vi "AI IRQ Config Pane.vi"(6 "_SubPanelMessages":refnum<notifier>, 9 "_myEmbeddedToFrameEvent":T7, 10 "_myEmbedded.Exit":refnum<user-event>, 11 "_Property Bundle":cluster{"Name":string, "Value":variant}[](array[cluster])) -> (1 "_Connection Informations":T2, 2 "_Scripter Input":T4)   [LabVIEW 2021]
doc: "Registers analog and digital input interrupts and creates timer interrupts."
uses:
  <vilib>/myRIO/Common/Express VI Framework/xctls/myRIO Channel Name/myRIO Channel Name.xctl
  <vilib>/myRIO/Common/Instrument Driver Framework/myRIO v1.0/IRQ/typedefs/AI IRQ Type.ctl
  <vilib>/myRIO/Common/Express VI Framework/typedefs/Config Pane to Framework Ref.ctl
  <vilib>/myRIO/Common/Express VI Framework/typedefs/Data Validate Ref.ctl
  <vilib>/myRIO/Common/Express VI Framework/typedefs/Sub Panel Messages.ctl
  <vilib>/myRIO/Common/Express VI Framework/typedefs/Instrument Driver Method Descriptor Array.ctl
  <vilib>/myRIO/Common/Express VI Framework/typedefs/Instrument Driver Method Descriptor.ctl
  <vilib>/myRIO/Common/Express VI Framework/typedefs/Scripter Input.ctl
  <vilib>/myRIO/Common/Express VI Framework/typedefs/WireThrough Terminal Names.ctl
  <vilib>/myRIO/Common/Express VI Framework/typedefs/Connection Informations.ctl
  <vilib>/myRIO/Common/Instrument Driver Framework/Utilities/typedefs/Channel Types.ctl
  <vilib>/myRIO/Common/Express VI Framework/vis/Express VI Framework Strings Global.vi
  <vilib>/myRIO/Express VI/IRQ/Message Globals.vi
panel:
  out "_create Callback?":bool
  in  "_Create Button":bool
  in  "Callback VI Path:":path
  out "_Warning Icon":picture
  out "_Error Message":string
  out "_Callback VI Path":string caption="Callback VI:"
  in  "_Open Button":bool
  out "_Hysteresis":string
  out "_Threhold":string
  out "_Analog Preview":T1(graph) caption="Preview:"
  in  "_callback":refnum<vi>
  in  "_VI Default Name (Edit and make value default)":string="Analog input interrupt"
  in  "_WireThrough Info (Edit and make value default)":T3={"WireThrough Top In"="Ref In", "WireThrough Bottom In"="error in (no error)", "WireThrough Top Out"="Ref Out", "WireThrough Bottom Out"="error out"}
  in  "_Template Array (Edit and make value default)":T5=[{"Function Name"="Register AI IRQ", "VI Path"=path "<vilib>/myRIO/Instrument Drivers/IRQ/IO IRQ/vis", "Script"=TRUE, "Inputs"=[{"name"="IRQ Number", "value"=variant, "Config Pane Only"=TRUE, "Build Array"=FALSE, "Bundle Cluster"=FALSE, "Show Term"=FALSE, "alias"=[], "Required Input"=FALSE}, {"name"="Analog Interrupt Type", "value"=variant, "Config Pane Only"=TRUE, "Build Array"=FALSE, "Bundle Cluster"=FALSE, "Show Term"=FALSE, "alias"=[], "Required Input"=FALSE}, {"name"="Channel Name", "value"=variant, "Config Pane Only"=TRUE, "Build Array"=FALSE, "Bundle Cluster"=FALSE, "Show Term"=FALSE, "alias"=[], "Required Input"=FALSE}, {"name"="Threshold", "value"=variant, "Config Pane Only"=TRUE, "Build Array"=FALSE, "Bundle Cluster"=FALSE, "Show Term"=FALSE, "alias"=[], "Required Input"=FALSE}, {"name"="Callback VI Reference", "value"=variant, "Config Pane Only"=FALSE, "Build Array"=FALSE, "Bundle Cluster"=FALSE, "Show Term"=TRUE, "alias"=[], "Required Input"=FALSE}], "Outputs"=[], "VI Class"=enum."Open", "Controls Refs[]"=[], "Inline"=FALSE}]
  in  "_Default Alias String":string
  in  "Type:":T9
  in  "Channel:":u16(xcontrol)
  in  "IRQ number:":u8 max=7
  in  "Threshold:":dbl=2.5 min=0.0 max=5.0
  in  "Name:":string="Analog input interrupt" caption="Node name:"
  out "_IRQ Learn More":string="The 0.02 hysteresis helps prevent multiple triggers due to noise."
  # "NOTE: Tab Order has been set\nfor this Front Panel.\n\nSee Edit>>Set Tabbing Order...\n\nAll controls that are not visible at \nruntime are excluded from Tabbing order\n\nTo exlude a control from context\nhelp prefix its label text with a '-'"
  # "Trigger point"
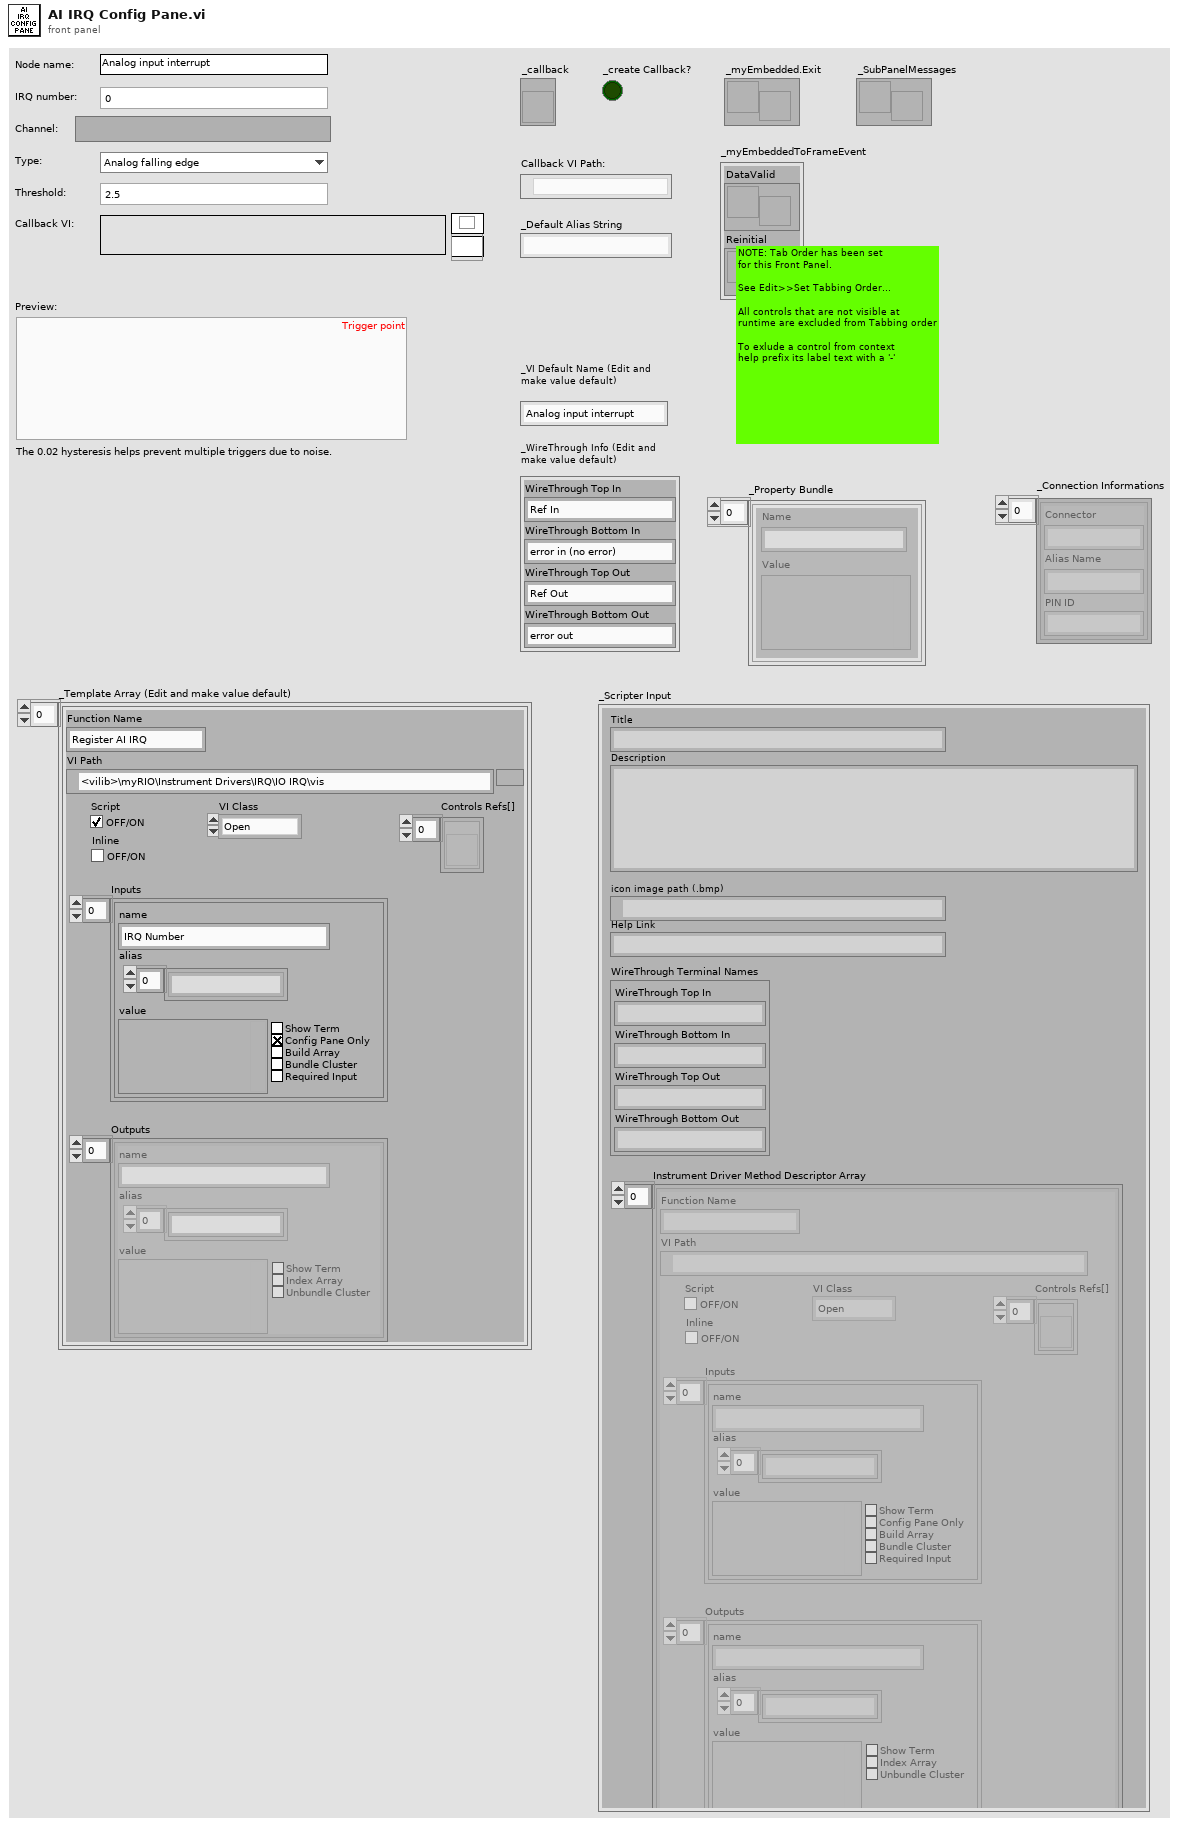
[diagram p1: front panel]
types:
  T1 = cluster{"Analog Preview 3":cluster{"X":dbl, "Y":dbl}[]}[]
  T2 = typedef "Connection Informations.ctl" = cluster{"Connector":string, "Alias Name":string, "PIN ID":string}[]
  T3 = typedef "WireThrough Terminal Names.ctl" = cluster{"WireThrough Top In":string, "WireThrough Bottom In":string, "WireThrough Top Out":string, "WireThrough Bottom Out":string}
  T4 = typedef "Scripter Input.ctl" = cluster{"Title":string, "Description":string, "icon image path (.bmp)":path, "Help Link":string, "WireThrough Terminal Names":T3, "Instrument Driver Method Descriptor Array":T5}
  T5 = typedef "Instrument Driver Method Descriptor Array.ctl" = T6[]
  T6 = typedef "Instrument Driver Method Descriptor.ctl" = cluster{"Function Name":string, "VI Path":path, "Script":bool, "Inputs":cluster{"name":string, "value":variant, "Config Pane Only":bool, "Build Array":bool, "Bundle Cluster":bool, "Show Term":bool, "alias":string[], "Required Input":bool}[], "Outputs":cluster{"name":string, "value":variant, "Show Term":bool, "Index Array":bool, "Unbundle Cluster":bool, "alias":string[]}[], "VI Class":enum16{"Open", "Configure", "Data", "Manage", "Close"}, "Controls Refs[]":refnum<vi>[], "Inline":bool}
  T7 = typedef "Config Pane to Framework Ref.ctl" = cluster{"DataValid":T8, "Reinitial":refnum<user-event>}
  T8 = typedef "Data Validate Ref.ctl" = refnum<user-event>
  T9 = typedef "AI IRQ Type.ctl" = enum16{"Analog falling edge", "Analog rising edge"}
  T10 = typedef "Channel Types.ctl" = enum32{"Unknown", "AI", "AO", "DIO - DI", "DIO", "DIO - DO", "I2C", "PWM", "Encoder", "SPI", "UART", "Accelerometer", "DIO - LED", "DIO - Button", "AI (N Samples)", "AudioIn (N Samples)", "AO (N Samples)", "AudioOut (N Samples)", "DI (N Samples)", "DO (N Samples)", "AI IRQ", "DI IRQ", "Timer IRQ", "RSL", "Relay", "CAN", "AI (Continuous)", "AO (Continuous)"}
  T11 = typedef "Channel Info.ctl" = cluster{"Channel Name":string, "Alias":string, "Used?":bool, "Not Support?":bool, "Property Bundle":cluster{"Name":string, "Value":variant}[]}
  T12 = typedef "Sub Panel Messages.ctl" = enum16{"Initialized"}
  T13 = cluster{"Connector":string, "Alias Name":string, "PIN ID":string}
  T14 = cluster{"left":i16, "top":i16, "right":i16, "bottom":i16}
  T15 = cluster{"name":string, "value":variant, "Config Pane Only":bool, "Build Array":bool, "Bundle Cluster":bool, "Show Term":bool, "alias":string[], "Required Input":bool}[]
  T16 = cluster{"name":string, "value":variant, "Config Pane Only":bool, "Build Array":bool, "Bundle Cluster":bool, "Show Term":bool, "alias":string[], "Required Input":bool}
  T17 = cluster{"Connector":string, "Alias Name":string, "PIN ID":string}[]
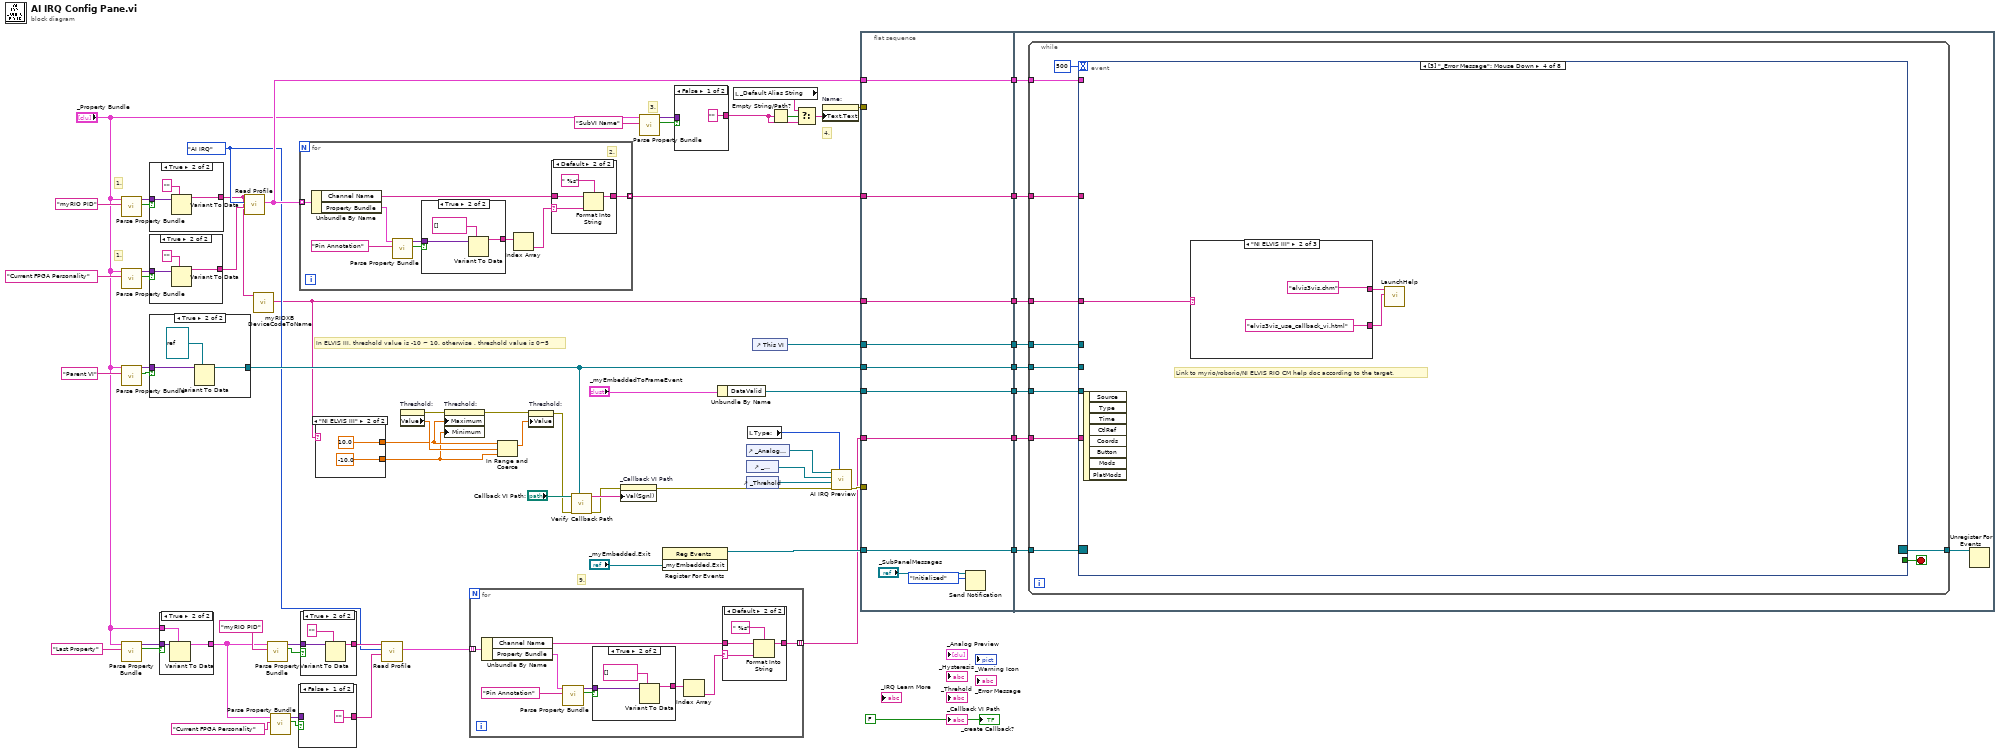
[diagram p0: block diagram]
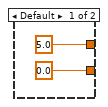
[diagram p2: hidden frame]
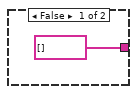
[diagram p3: hidden frame]
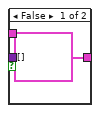
[diagram p5: hidden frame]
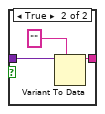
[diagram p6: hidden frame]
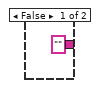
[diagram p7: hidden frame]
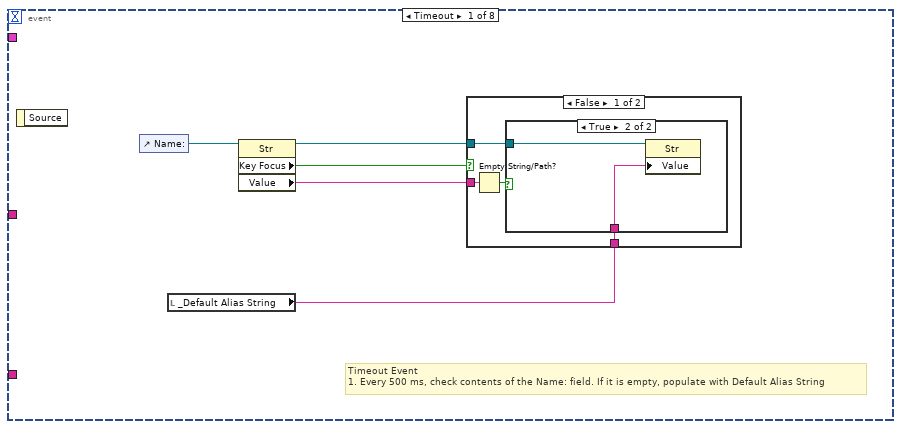
[diagram p8: hidden frame]
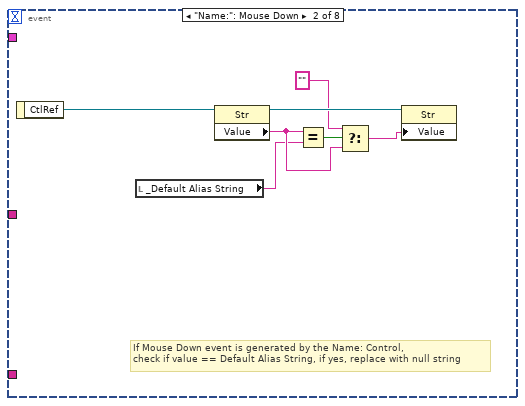
[diagram p11: hidden frame]
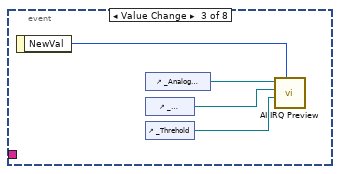
[diagram p12: hidden frame]
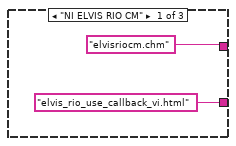
[diagram p13: hidden frame]
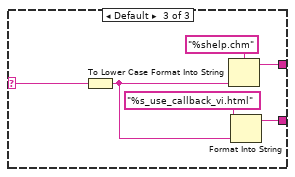
[diagram p14: hidden frame]
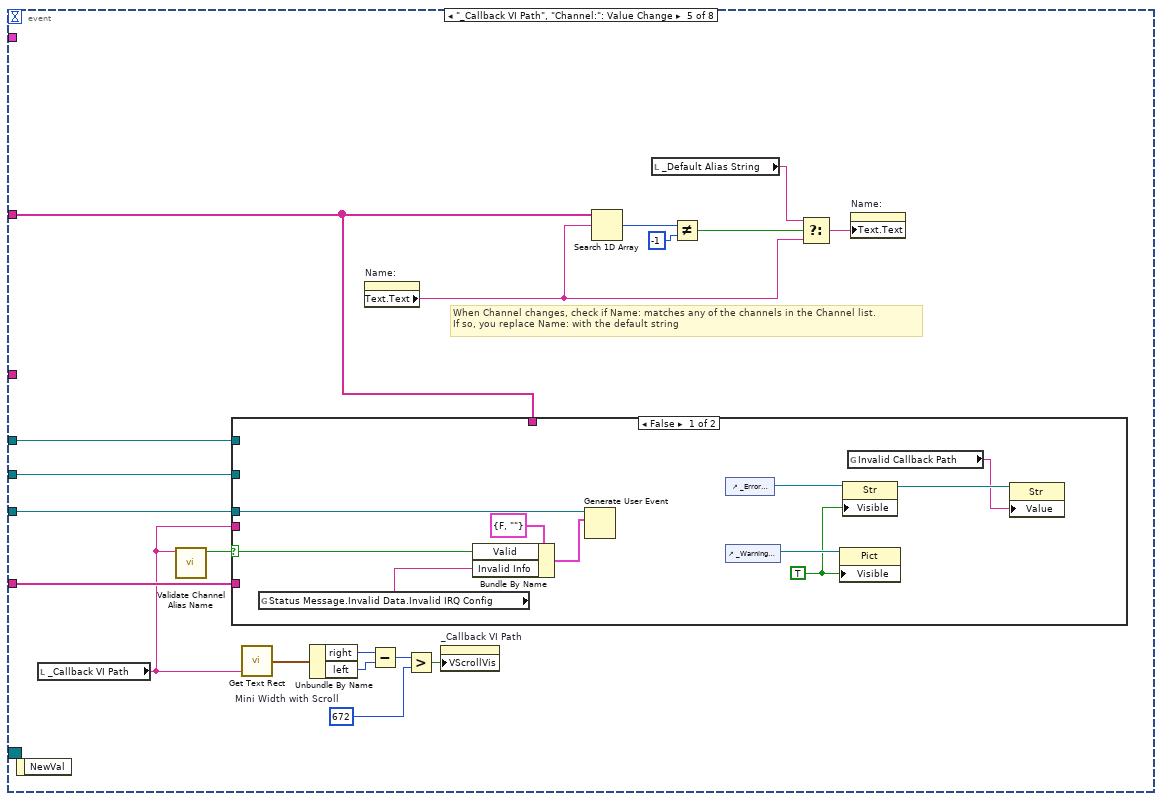
[diagram p15: hidden frame]
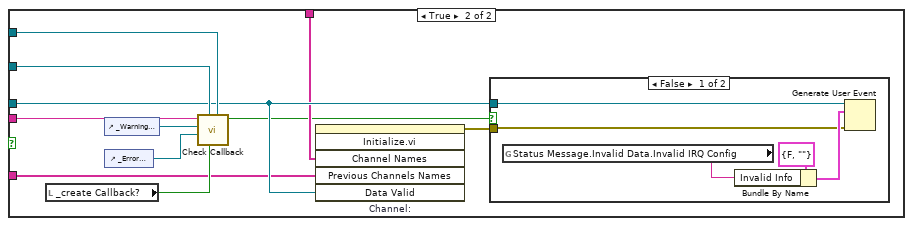
[diagram p16: hidden frame]
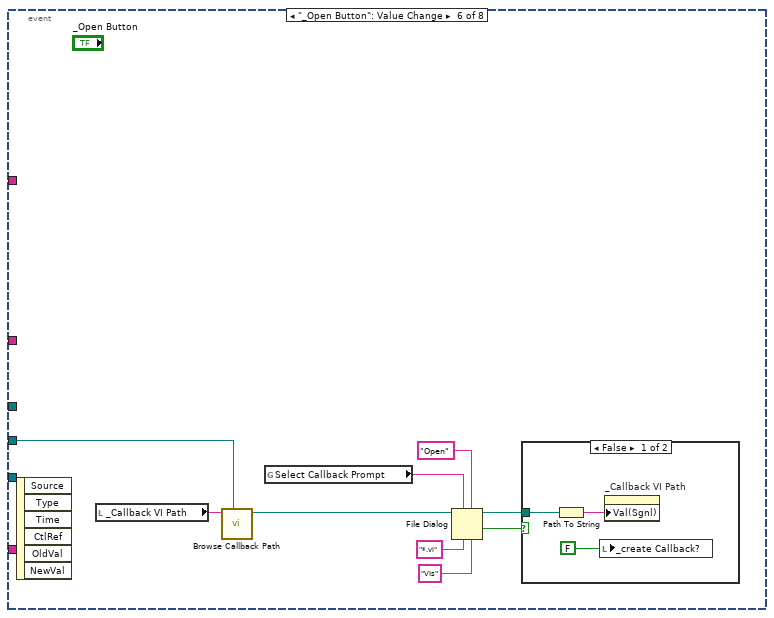
[diagram p18: hidden frame]
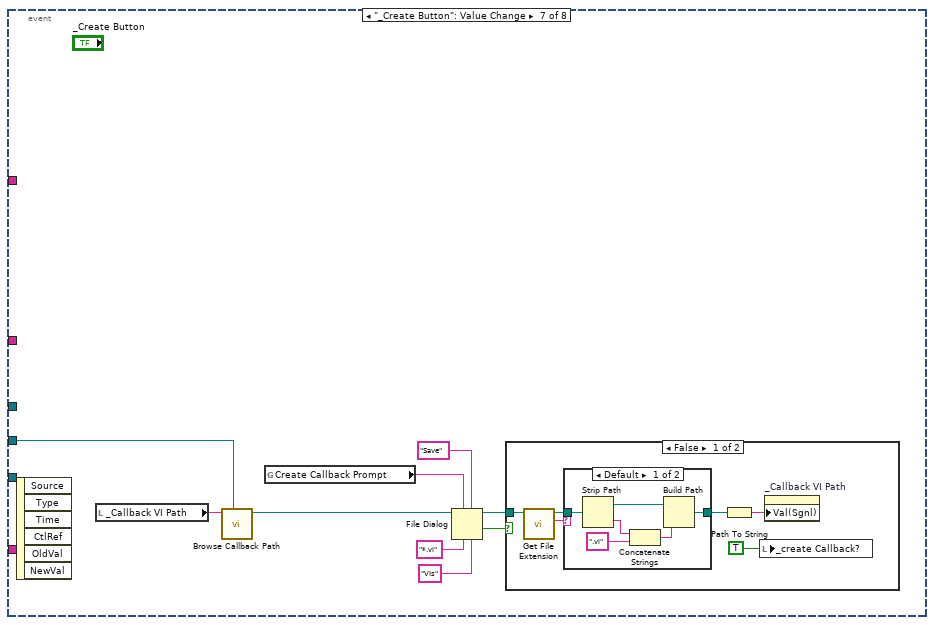
[diagram p20: hidden frame]
diagram:
  w15 = Channel_Types."AI IRQ" ("Channel to Read")
  # "In ELVIS III, threshold value is -10 ~ 10. otherwise , threshold value is 0~5"
  # "1."
  # "1."
  # "9."
  # "4."
  # "3."
  n1 = call <vilib>:"Parse Property Bundle.vi"("Name"="myRIO PID", "Property Bundle"="_Property Bundle") -> ("Found?"=w61:bool, "Value"=w62:variant)  [unwired: 8 in]
  n2 = call <vilib>:"Parse Property Bundle.vi"("Name"="Current FPGA Personality", "Property Bundle"="_Property Bundle") -> ("Found?"=w60:bool, "Value"=w59:variant)  [unwired: 8 in]
  n3 = call <vilib>:"Parse Property Bundle.vi"("Name"="Parent VI", "Property Bundle"="_Property Bundle") -> ("Found?"=w52:bool, "Value"=w51:variant)  [unwired: 8 in]
  n4 = call <vilib>:"Parse Property Bundle.vi"("Name"="Last Property", "Property Bundle"="_Property Bundle") -> ("Found?"=w18:bool, "Value"=w19:variant)  [unwired: 8 in]
  n5 = case shown="True" w61 {
    tunnel: w62 -> [_ w73]
    tunnel: ["" ("Name") w71] -> w9
    frame False {
    }
    frame True {
      n6 = Variant To Data(type="" ("Name"), Variant=w73) -> (data=w71:string)  [unwired: 1 in, 1 out]
    }
  }
  n7 = case shown="True" w60 {
    tunnel: w59 -> [_ w77]
    tunnel: ["" ("Name") w75] -> w57
    frame False {
    }
    frame True {
      n8 = Variant To Data(type="" ("Name"), Variant=w77) -> (data=w75:string)  [unwired: 1 in, 1 out]
    }
  }
  n9 = case shown="True" w52 {
    tunnel: w51 -> [_ w81]
    tunnel: [refnum<vi> refnum ("reference out") w79] -> w45
    frame False {
    }
    frame True {
      n10 = Variant To Data(type=refnum<vi> refnum ("reference out"), Variant=w81) -> (data=w79:refnum<vi>)  [unwired: 1 in, 1 out]
    }
  }
  n11 = case shown="True" w18 {
    tunnel: w19 -> [_ w85]
    tunnel: [cluster{"Name":string, "Value":variant}[] [] ("_Property Bundle") w84] -> w17
    tunnel: "_Property Bundle" -> [_ w83]
    frame False {
    }
    frame True {
      n12 = Variant To Data(type=w83, Variant=w85) -> (data=w84:cluster{"Name":string, "Value":variant}[])  [unwired: 1 in, 1 out]
    }
  }
  n13 = call <vilib>:"Read Profile.vi"("FPGA Name"=w57, "Channel to Read"=w15, "myRIO PID"=w9) -> ("Channel List Out"=w55:T11[])  [unwired: 7 in, 1 out]
  n14 = call <vilib>:"myRIOXB DeviceCodeToName.vi"("Device Code"=w9) -> ("Name"=w8:string)  [unwired: 10 in]
  n15 = call <vilib>:"Parse Property Bundle.vi"("Name"="myRIO PID", "Property Bundle"=w17) -> ("Found?"=w27:bool, "Value"=w26:variant)  [unwired: 8 in]
  n16 = call <vilib>:"Parse Property Bundle.vi"("Name"="Current FPGA Personality", "Property Bundle"=w17) -> ("Found?"=w22:bool, "Value"=w23:variant)  [unwired: 8 in]
  n17 = case shown="False" w22 {
    tunnel: w23 -> [_ w89]
    tunnel: ["" ("Name") w87] -> w21
    frame False {
    }
    frame True {
      n18 = Variant To Data(type="" ("Name"), Variant=w89) -> (data=w87:string)  [unwired: 1 in, 1 out]
    }
  }
  n19 = for {
    tunnel: w55 -> [w97] mode=indexing
    tunnel: [w98] -> w29 mode=indexing
    # "2."
    n20 = Unbundle By Name(w97) -> ("Channel Name"=w96:string, "Property Bundle"=w95:cluster{"Name":string, "Value":variant}[])
    n21 = call <vilib>:"Parse Property Bundle.vi"("Name"="Pin Annotation", "Property Bundle"=w95) -> ("Found?"=w92:bool, "Value"=w93:variant)  [unwired: 8 in]
    n22 = case shown="True" w92 {
      tunnel: w93 -> [_ w102]
      tunnel: [string[] [] w101] -> w91
      frame False {
      }
      frame True {
        n23 = Variant To Data(type=string[] [], Variant=w102) -> (data=w101:string[])  [unwired: 1 in, 1 out]
      }
    }
    n24 = Index Array(array=w91) -> (element=w90:string)  [unwired: 1 in]
    n25 = case shown="Default" w90 {
      selector: w90 -> [_ w106]
      tunnel: w96 -> [w103 w105]
      tunnel: [w103 w104] -> w98
      frame "" {
      }
      frame Default {
        n26 = Format Into String(format string=" %s", initial string=w105, w106) -> (resulting string=w104:string)  [unwired: 1 in, 1 out]
      }
    }
  }
  n27 = case shown="True" w27 {
    tunnel: w26 -> [_ w111]
    tunnel: ["" ("Name") w109] -> w28
    frame False {
    }
    frame True {
      n28 = Variant To Data(type="" ("Name"), Variant=w111) -> (data=w109:string)  [unwired: 1 in, 1 out]
    }
  }
  n29 = case shown="\"NI ELVIS III\"" w8 {
    tunnel: [5.0 ("Data Entry Limits:Maximum") 10.0 ("Data Entry Limits:Maximum")] -> w6
    tunnel: [0.0 -10.0] -> w5
    frame Default {
    }
    frame "NI ELVIS III" {
    }
  }
  n30 = call <vilib>:"Read Profile.vi"("FPGA Name"=w21, "Channel to Read"=w15, "myRIO PID"=w28) -> ("Channel List Out"=w13:T11[])  [unwired: 7 in, 1 out]
  n31 = property on="Threshold:" class="DigNum (strict)"() -> (error out=w3:errorcluster, "Value"=w7:dbl)  [unwired: 2 in, 1 out]
  n32 = property on="Threshold:" class="DigNum (strict)"(error in=w3, "Maximum"=w6, "Minimum"=w5) -> (error out=w2:errorcluster)  [unwired: 1 in, 1 out]
  n33 = for {
    tunnel: w13 -> [w123] mode=indexing
    tunnel: [w124] -> w12 mode=indexing
    n34 = Unbundle By Name(w123) -> ("Channel Name"=w122:string, "Property Bundle"=w121:cluster{"Name":string, "Value":variant}[])
    n35 = call <vilib>:"Parse Property Bundle.vi"("Name"="Pin Annotation", "Property Bundle"=w121) -> ("Found?"=w118:bool, "Value"=w119:variant)  [unwired: 8 in]
    n36 = case shown="True" w118 {
      tunnel: w119 -> [_ w128]
      tunnel: [string[] [] w127] -> w117
      frame False {
      }
      frame True {
        n37 = Variant To Data(type=string[] [], Variant=w128) -> (data=w127:string[])  [unwired: 1 in, 1 out]
      }
    }
    n38 = Index Array(array=w117) -> (element=w116:string)  [unwired: 1 in]
    n39 = case shown="Default" w116 {
      selector: w116 -> [_ w132]
      tunnel: w122 -> [w129 w131]
      tunnel: [w129 w130] -> w124
      frame "" {
      }
      frame Default {
        n40 = Format Into String(format string=" %s", initial string=w131, w132) -> (resulting string=w130:string)  [unwired: 1 in, 1 out]
      }
    }
  }
  n41 = In Range and Coerce(upper limit=w6, x=w7, lower limit=w5) -> (coerced(x)=w4:dbl)  [unwired: 1 out]
  n42 = property on="Threshold:" class="DigNum (strict)"(error in=w2, "Value"=w4) -> (error out=w1:errorcluster)  [unwired: 1 in, 1 out]
  n43 = call <vilib>:"Verify Callback Path.vi"("Parent VI Ref"=w45, "error in (no error)"=w1, "Saved Callback Path"="Callback VI Path:") -> ("error out"=w42:errorcluster, "Valid Path out"=w43:string)  [unwired: 7 in]
  n44 = property on="_Callback VI Path" class="Str"(error in=w42, "Val(Sgnl)"=w43) -> (error out=w41:errorcluster)  [unwired: 1 in, 1 out]
  n45 = call <vilib>:"Parse Property Bundle.vi"("Name"="SubVI Name", "Property Bundle"="_Property Bundle") -> ("Found?"=w66:bool, "Value"=w65:variant)  [unwired: 8 in]
  n46 = register-events("_myEmbedded.Exit") -> (reference out=w56:refnum<event-registration>)  [unwired: 2 in, 1 out]
  n47 = case shown="False" w66 {
    tunnel: w65 -> [_ w137]
    tunnel: ["" ("Name") w135] -> w64
    frame False {
    }
    frame True {
      n48 = Variant To Data(type="" ("Name"), Variant=w137) -> (data=w135:string)  [unwired: 1 in, 1 out]
    }
  }
  n49 = Unbundle By Name("_myEmbeddedToFrameEvent") -> ("DataValid"=w37:T8)
  n50 = local read "_Default Alias String"() -> (w54:string)
  n51 = control-ref of="_Analog Preview"() -> (w47:refnum<vi>)
  n52 = control-ref of="_Hysteresis"() -> (w48:refnum<vi>)
  n53 = control-ref of="_Threhold"() -> (w49:refnum<vi>)
  n54 = local read "Type:"() -> (w46:T9)
  n55 = control-ref of="This VI"() -> (w44:refnum<vi>)
  n56 = Empty String/Path?(string/path=w64) -> (empty?=w68:bool)
  n57 = Select(t=w54, s=w68, f=w64) -> (s? t:f=w53:string)
  n58 = property on="Name:" class="Str"("Text.Text"=w53) -> (error out=w10:errorcluster)  [unwired: 2 in, 1 out]
  n59 = call <vilib>:"AI IRQ Preview.vi"("Type"=w46, "error in (no error)"=w41, "_Threhold Refnum"=w49, "_Hysteresis Refnum"=w48, "_Analog Preview Refnum"=w47) -> ("error out"=w39:errorcluster)  [unwired: 6 in]
  n60 = flat-sequence {
    tunnel: w37 -> [w139]
    tunnel: w39 -> [_]
    tunnel: w44 -> [w144]
    tunnel: w45 -> [w145]
    tunnel: w55 -> [w146]
    tunnel: w56 -> [w140]
    tunnel: [w140] -> w36
    tunnel: [w146] -> w35
    tunnel: [w145] -> w34
    tunnel: [w144] -> w33
    tunnel: [w139] -> w32
    tunnel: [w141] -> w30
    tunnel: w8 -> [w141]
    tunnel: w29 -> [w147]
    tunnel: w12 -> [w138]
    tunnel: [w147] -> w14
    tunnel: [w138] -> w11
    tunnel: w10 -> [_]
    tunnel: w36 -> [w156]
    tunnel: w35 -> [w155]
    tunnel: w34 -> [w153]
    tunnel: w33 -> [w152]
    tunnel: w32 -> [w151]
    tunnel: w30 -> [w150]
    tunnel: w14 -> [w149]
    tunnel: w11 -> [w148]
    frame #0 {
      n61 = Send Notification(notification=Sub_Panel_Messages."Initialized", notifier="_SubPanelMessages") -> ()  [unwired: 1 in, 2 out]
    }
    frame #1 {
      n62 = while {
        tunnel: w156 -> [w166]
        tunnel: w151 -> [w158]
        tunnel: w155 -> [w163]
        tunnel: [w164] -> w154
        tunnel: w153 -> [w162]
        tunnel: w152 -> [w161]
        tunnel: w150 -> [w160]
        tunnel: w149 -> [w159]
        tunnel: w148 -> [w157]
        stop <- w165 stop-if-true
        n63 = event shown="[3] \"_Error Message\": Mouse Down" {
          selector: w166 -> [_ _ _ _ _ _ _ _]
          dyn-events: [_ _ _ _ _ _ _ _] -> w164
          timeout: 500 -> [_ _ _ _ _ _ _ _]
          tunnel: [_ _ _ _ _ _ _ TRUE ("Valid Callback?")] -> w165
          tunnel: w163 -> [_ _ _ _ _ _ _ w325]
          tunnel: w158 -> [_ _ _ _ w207 _ _ _]
          tunnel: w162 -> [_ _ _ _ w221 w248 w260 w285]
          tunnel: w161 -> [_ _ _ _ w220 _ _ _]
          tunnel: w160 -> [_ _ _ w190 _ _ _ _]
          tunnel: w159 -> [_ _ _ _ w206 _ _ _]
          tunnel: w157 -> [_ _ _ _ w205 _ _ _]
          event Timeout {
            # "Timeout Event\n1. Every 500 ms, check contents of the Name: field. If it is empty, populate with Default Alias String"
            n64 = event-data() -> ()  [unwired: 1 in, 1 out]
            n65 = control-ref of="Name:"() -> (w169:refnum<vi>)
            n66 = local read "_Default Alias String"() -> (w168:string)
            n67 = property on="Property Node" class="Str"(reference=w169) -> (reference out=w172:refnum<vi>, "Key Focus"=w171:bool, "Value"=w170:string)  [unwired: 1 in, 1 out]
            n68 = case shown="False" w171 {
              tunnel: w170 -> [w176 _]
              tunnel: w172 -> [w174 _]
              tunnel: w168 -> [w173 _]
              frame False {
                n69 = Empty String/Path?(string/path=w176) -> (empty?=w175:bool)
                n70 = case shown="True" w175 {
                  tunnel: w174 -> [_ w178]
                  tunnel: w173 -> [_ w177]
                  frame False {
                  }
                  frame True {
                    n71 = property on="Property Node" class="Str"(reference=w178, "Value"=w177) -> ()  [unwired: 1 in, 2 out]
                  }
                }
              }
              frame True {
              }
            }
          }
          event "Name:": Mouse Down {
            # "If Mouse Down event is generated by the Name: Control,\ncheck if value == Default Alias String, if yes, replace with null string"
            n72 = event-data() -> ("CtlRef"=w180:refnum<vi>)  [unwired: 1 in]
            n73 = local read "_Default Alias String"() -> (w179:string)
            n74 = property class="Str"(reference=w180) -> (reference out=w184:refnum<vi>, "Value"=w185:string)  [unwired: 1 in, 1 out]
            n75 = Equal?(x=w185, y=w179) -> (x = y?=w181:bool)
            n76 = Select(t="", s=w181, f=w185) -> (s? t:f=w183:string)
            n77 = property class="Str"(reference=w184, "Value"=w183) -> ()  [unwired: 1 in, 2 out]
          }
          event Value Change {
            n78 = event-data() -> ("NewVal"=w186:T9)  [unwired: 1 in]
            n79 = control-ref of="_Analog Preview"() -> (w189:refnum<vi>)
            n80 = control-ref of="_Hysteresis"() -> (w188:refnum<vi>)
            n81 = control-ref of="_Threhold"() -> (w187:refnum<vi>)
            n82 = call <vilib>:"AI IRQ Preview.vi"("Type"=w186, "_Threhold Refnum"=w187, "_Hysteresis Refnum"=w188, "_Analog Preview Refnum"=w189) -> ()  [unwired: 7 in, 1 out]
          }
          event "_Error Message": Mouse Down {
            # "Link to myrio/roborio/NI ELVIS RIO CM help doc according to the target."
            n83 = event-data() -> ()  [unwired: 1 in, 8 out]
            n84 = case shown="\"NI ELVIS III\"" w190 {
              selector: w190 -> [_ _ w197]
              tunnel: ["elvisriocm.chm" ("Help File") "elvis3vis.chm" ("Help File") w199] -> w192
              tunnel: ["elvis_rio_use_callback_vi.html" ("Help Topic") "elvis3vis_use_callback_vi.html" ("Help Topic") w198] -> w191
              frame "NI ELVIS RIO CM" {
              }
              frame "NI ELVIS III" {
              }
              frame Default {
                n85 = To Lower Case(string=w197) -> (all lower case string=w201:string)
                n86 = Format Into String(format string="%shelp.chm" ("Help File"), w201) -> (resulting string=w199:string)  [unwired: 2 in, 1 out]
                n87 = Format Into String(format string="%s_use_callback_vi.html" ("Help Topic"), w201) -> (resulting string=w198:string)  [unwired: 2 in, 1 out]
              }
            }
            n88 = call <vilib>:"LaunchHelp.vi"("Help Topic"=w191, "Help File"=w192) -> ()  [unwired: 10 in]
          }
          event "_Callback VI Path", "Channel:": Value Change {
            w215 = i16 672  # Mini Width with Scroll
            # "When Channel changes, check if Name: matches any of the channels in the Channel list. \nIf so, you replace Name: with the default string"
            n89 = event-data() -> ()  [unwired: 1 in, 1 out]
            n90 = local read "_Callback VI Path"() -> (w204:string)
            n91 = call <vilib>:"Validate Channel Alias Name.vi"("Channel Alias"=w204) -> ("Valid?"=w203:bool)  [unwired: 9 in, 1 out]
            n92 = case shown="False" w203 {
              selector: w203 -> [w228 _]
              tunnel: w221 -> [_ w241]
              tunnel: w220 -> [_ w238]
              tunnel: w204 -> [_ w236]
              tunnel: w207 -> [w229 w235]
              tunnel: w206 -> [_ w234]
              tunnel: w205 -> [_ w233]
              frame False {
                w225 = TRUE ("Visible")
                n93 = global read "Express VI Framework Strings Global.vi" "Status Message.Invalid Data.Invalid IRQ Config"() -> (w224:string)
                n94 = Bundle By Name(cluster=cluster{"Valid":bool, "Invalid Info":string} {"Valid"=FALSE, "Invalid Info"=""} ("event data"), "Valid"=w228, "Invalid Info"=w224) -> (w231:cluster{"Valid":bool, "Invalid Info":string})
                n95 = Generate User Event(user event=w229, event data cluster=w231) -> ()  [unwired: 2 in, 2 out]
                n96 = control-ref of="_Error Message"() -> (w226:refnum<vi>)
                n97 = control-ref of="_Warning Icon"() -> (w227:refnum<vi>)
                n98 = property class="Pict"(reference=w227, "Visible"=w225) -> ()  [unwired: 1 in, 2 out]
                n99 = property class="Str"(reference=w226, "Visible"=w225) -> (reference out=w223:refnum<vi>)  [unwired: 1 in, 1 out]
                n100 = global read "Message Globals.vi" "Invalid Callback Path"() -> (w222:string)
                n101 = property class="Str"(reference=w223, "Value"=w222) -> ()  [unwired: 1 in, 2 out]
              }
              frame True {
                n102 = local read "_create Callback?"() -> (w237:bool)
                n103 = control-ref of="_Warning Icon"() -> (w240:refnum<vi>)
                n104 = control-ref of="_Error Message"() -> (w239:refnum<vi>)
                n105 = call <vilib>:"Check Callback.vi"("Config VI Ref"=w238, "Create Callback?"=w237, "Parent VI Ref"=w241, "Error Message Ref"=w239, "Warning Icon Ref"=w240, "Callback Path"=w236) -> ("Valid Callback?"=w232:bool)  [unwired: 5 in]
                n106 = invoke on="Channel:" class="myRIO Channel Name (strict)" method="Initialize.vi"("Channel Names"=w234, "Previous Channels Names"=w233, "Data Valid"=w235) -> (error out=w242:errorcluster)  [unwired: 3 in, 5 out]
                n107 = case shown="False" w232 {
                  tunnel: w235 -> [w245 _]
                  tunnel: w242 -> [w243 _]
                  frame False {
                    n108 = global read "Express VI Framework Strings Global.vi" "Status Message.Invalid Data.Invalid IRQ Config"() -> (w244:string)
                    n109 = Bundle By Name(cluster=cluster{"Valid":bool, "Invalid Info":string} {"Valid"=FALSE, "Invalid Info"=""} ("event data"), "Invalid Info"=w244) -> (w247:cluster{"Valid":bool, "Invalid Info":string})
                    n110 = Generate User Event(user event=w245, event data cluster=w247, error in=w243) -> ()  [unwired: 1 in, 2 out]
                  }
                  frame True {
                  }
                }
              }
            }
            n111 = call <vilib>:"Get Text Rect.vi"("text"=w204) -> ("rect"=w219:T14)  [unwired: 8 in]
            n112 = Unbundle By Name(w219) -> ("right"=w218:i16, "left"=w217:i16)
            n113 = property on="Name:" class="Str"() -> ("Text.Text"=w209:string)  [unwired: 2 in, 2 out]
            n114 = Subtract(x=w218, y=w217) -> (x-y=w216:i16)
            n115 = Greater?(x=w216, y=w215) -> (0:w214:bool)
            n116 = property on="_Callback VI Path" class="Str"("VScrollVis"=w214) -> ()  [unwired: 2 in, 2 out]
            n117 = Search 1D Array(1D array=w206, element=w209) -> (index of element=w212:i32)  [unwired: 1 in]
            n118 = local read "_Default Alias String"() -> (w211:string)
            n119 = Not Equal?(x=w212, y=-1) -> (x != y?=w213:bool)
            n120 = Select(t=w211, s=w213, f=w209) -> (s? t:f=w210:string)
            n121 = property on="Name:" class="Str"("Text.Text"=w210) -> ()  [unwired: 2 in, 2 out]
          }
          event "_Open Button": Value Change {
            n122 = event-data() -> ()  [unwired: 1 in, 6 out]
            n123 = local read "_Callback VI Path"() -> (w250:string)
            n124 = call <vilib>:"Browse Callback Path.vi"("Parent VI Ref"=w248, "Init Path in"=w250) -> ("Init Path out"=w249:path)  [unwired: 9 in]
            n125 = global read "Message Globals.vi" "Select Callback Prompt"() -> (w252:string)
            n126 = File Dialog(4:"VIs" ("pattern label"), 5:"Open" ("button label"), 6:"*.vi" ("pattern (all files)"), 7:w252, 11:w249) -> (1:w255:bool, 3:w256:path)  [unwired: 2 in, 2 out]
            n127 = case shown="False" w255 {
              tunnel: w256 -> [w259 _]
              frame False {
                n128 = Path To String(path=w259) -> (string=w258:string)
                n129 = local write "_create Callback?"(FALSE ("_new Callback?")) -> ()
                n130 = property on="_Callback VI Path" class="Str"("Val(Sgnl)"=w258) -> ()  [unwired: 2 in, 2 out]
              }
              frame True {
              }
            }
          }
          event "_Create Button": Value Change {
            n131 = event-data() -> ()  [unwired: 1 in, 6 out]
            n132 = local read "_Callback VI Path"() -> (w262:string)
            n133 = call <vilib>:"Browse Callback Path.vi"("Parent VI Ref"=w260, "Init Path in"=w262) -> ("Init Path out"=w261:path)  [unwired: 9 in]
            n134 = global read "Message Globals.vi" "Create Callback Prompt"() -> (w264:string)
            n135 = File Dialog(4:"VIs" ("pattern label"), 5:"Save" ("button label"), 6:"*.vi" ("pattern (all files)"), 7:w264, 11:w261) -> (1:w267:bool, 3:w268:path)  [unwired: 2 in, 2 out]
            n136 = case shown="False" w267 {
              tunnel: w268 -> [w270 _]
              frame False {
                n137 = call <vilib>:"Get File Extension.vi"("file"=w270) -> ("lowercase file extension"=w271:string, "dup file"=w272:path)  [unwired: 6 in, 3 out]
                n138 = case shown="Default" w271 {
                  tunnel: w272 -> [w280 w281]
                  tunnel: [w276 w281] -> w269
                  frame Default {
                    n139 = Strip Path(path=w280) -> (stripped path=w279:path, name=w278:string)
                    n140 = Concatenate Strings(w278, ".vi" ("string")) -> (w277:string)
                    n141 = Build Path(base path=w279, name or relative path=w277) -> (appended path=w276:path)
                  }
                  frame "vi" {
                  }
                }
                n142 = Path To String(path=w269) -> (string=w274:string)
                n143 = local write "_create Callback?"(TRUE ("_new VI")) -> ()
                n144 = property on="_Callback VI Path" class="Str"("Val(Sgnl)"=w274) -> ()  [unwired: 2 in, 2 out]
              }
              frame True {
              }
            }
          }
          event User Event {
            w309 = 0
            n145 = event-data() -> ("myEmbedded.Exit"=w282:bool)  [unwired: 1 in]
            n146 = property on="_Callback VI Path" class="Str"() -> ("Value"=w284:string)  [unwired: 2 in, 2 out]
            n147 = case shown="True" w282 {
              tunnel: w285 -> [_ w333]
              tunnel: w284 -> [w327 w331]
              tunnel: [w327 w330] -> w283
              frame False {
              }
              frame True {
                n148 = local read "_create Callback?"() -> (w329:bool)
                n149 = vi-ref <vilib>:"IO IRQ Callback .vit"() -> (w328:refnum<vi>)
                n150 = call <vilib>:"Create Callback.vi"("Create Callback?"=w329, "Parent VI Ref"=w333, "Template VI Ref"=w328, "Callback Path"=w331) -> ("Saved Callback Path"=w332:path, "Dup Callback Path"=w330:string)  [unwired: 6 in]
                n151 = local write "Callback VI Path:"(w332) -> ()
              }
            }
            n152 = Index Array(array=w325, index="Channel:") -> (element=w326:T11)
            n153 = Unbundle By Name(w326) -> ("Channel Name"=w300:string, "Property Bundle"=w296:cluster{"Name":string, "Value":variant}[])
            n154 = Build Array(w283) -> (w308:string[])
            n155 = in-place {
              in-place-border: "IRQ number:" -> [w341]
              in-place-border: "Type:" -> [w340]
              in-place-border: w300 -> [w339]
              in-place-border: "Threshold:" -> [w338]
              in-place-border: "_callback" -> [w337]
              in-place-border: w309 -> [w335]
              in-place-border: w308 -> [w334]
              n156 = in-place-array #1("_Template Array (Edit and make value default)", w309) -> (w342:T6)
              n157 = in-place {
                in-place-border: w341 -> [w354]
                in-place-border: w340 -> [w353]
                in-place-border: w339 -> [w352]
                in-place-border: w338 -> [w351]
                in-place-border: w337 -> [w350]
                in-place-border: w335 -> [w343]
                in-place-border: w334 -> [w344]
                n158 = in-place-cluster #2(w342) -> ("Inputs"=w355:T15)
                n159 = in-place {
                  in-place-border: w354 -> [w368]
                  in-place-border: w353 -> [w367]
                  in-place-border: w352 -> [w366]
                  in-place-border: w351 -> [w365]
                  in-place-border: w350 -> [w364]
                  in-place-border: w344 -> [w356]
                  n160 = in-place-array #3(w355, w343, 1, 2, 3, 4) -> (w371:T16, w370:T16, w369:T16, w363:T16, w362:T16)
                  n161 = Bundle By Name(cluster=w371, "value"=w368) -> (w357:T16)
                  n162 = Bundle By Name(cluster=w370, "value"=w367) -> (w358:T16)
                  n163 = Bundle By Name(cluster=w369, "value"=w366) -> (w359:T16)
                  n164 = Bundle By Name(cluster=w363, "value"=w365) -> (w360:T16)
                  n165 = Bundle By Name(cluster=w362, "value"=w364, "alias"=w356) -> (w361:T16)
                  n166 = in-place-array #3(w357, w358, w359, w360, w361) -> (w349:T15)  [unwired: 5 out]
                }
                n167 = in-place-cluster #2("Inputs"=w349) -> (w336:T6)
              }
              n168 = in-place-array #1(w336) -> (w315:T5)  [unwired: 1 out]
            }
            n169 = call <vilib>:"Parse Property Bundle.vi"("Name"="Pin Annotation" ("x"), "Property Bundle"=w296) -> ("Value"=w295:variant)  [unwired: 8 in, 1 out]
            n170 = Variant To Data(type=string[] [], Variant=w295) -> (data=w297:string[])  [unwired: 1 in, 1 out]
            n171 = Index Array(array=w297) -> (element=w288:string)  [unwired: 1 in]
            n172 = Match Pattern(string=w300, regular expression="/") -> (before substring=w302:string, after substring=w305:string)  [unwired: 1 in, 2 out]
            n173 = call <vilib>:"Trim Whitespace.vi"("string"=w305) -> ("trimmed string"=w306:string)  [unwired: 1 in]
            n174 = Match Pattern(string=w288, regular expression="(") -> (after substring=w290:string)  [unwired: 1 in, 3 out]
            n175 = Equal?(x="_Default Alias String", y="Name:") -> (x = y?=w318:bool)
            n176 = Concatenate Strings("Connector " ("string"), w302) -> (w303:string)
            n177 = Match Pattern(string=w290, regular expression=")") -> (before substring=w287:string)  [unwired: 1 in, 3 out]
            n178 = Select(t="_VI Default Name (Edit and make value default)", s=w318, f="Name:") -> (s? t:f=w319:string)
            n179 = Bundle By Name(cluster=T13 {"Connector"="", "Alias Name"="", "PIN ID"=""} ("Connection Information"), "Connector"=w303, "Alias Name"=w306, "PIN ID"=w287) -> (w299:T13)
            n180 = Bundle By Name(cluster=T4 {"Title"="", "Description"="", "icon image path (.bmp)"=path "", "Help Link"="", "WireThrough Terminal Names"={"WireThrough Top In"="", "WireThrough Bottom In"="", "WireThrough Top Out"="", "WireThrough Bottom Out"=""}, "Instrument Driver Method Descriptor Array"=[]} ("Scripter Input"), "Instrument Driver Method Descriptor Array"=w315, "WireThrough Terminal Names"="_WireThrough Info (Edit and make value default)", "Title"=w319, "Description"="" ("Title")) -> (→"_Scripter Input":T4)
            n181 = Build Array(w299) -> (→"_Connection Informations":T17)
          }
        }
      }
      n182 = Unregister For Events(event registration refnum=w154) -> ()  [unwired: 1 in, 1 out]
    }
  }
  "_create Callback?" <- FALSE ("_new VI")
